vi "Shoot-Vision.vi"(11 "VisionDistance":dbl) -> (1 "Possible":bool, 2 "Speed":dbl, 3 "Angle":dbl)   [LabVIEW 2019]
panel:
  in  "maxVelocity":dbl=10.0
  in  "V2":dbl
  in  "V1":dbl
  in  "distanceToTarget":dbl
  in  "targetHight":dbl=280.0
  in  "gravityConst":dbl=9.8
  in  "angle 2":dbl=60.0
  in  "angle 1":dbl=30.0
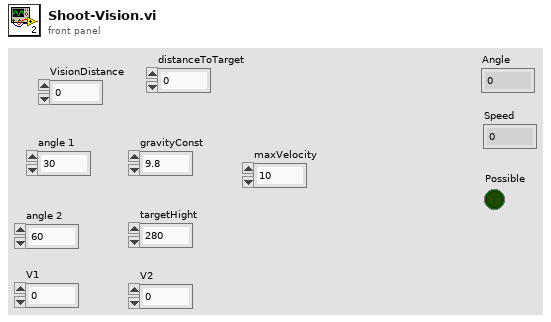
[diagram p1: front panel]
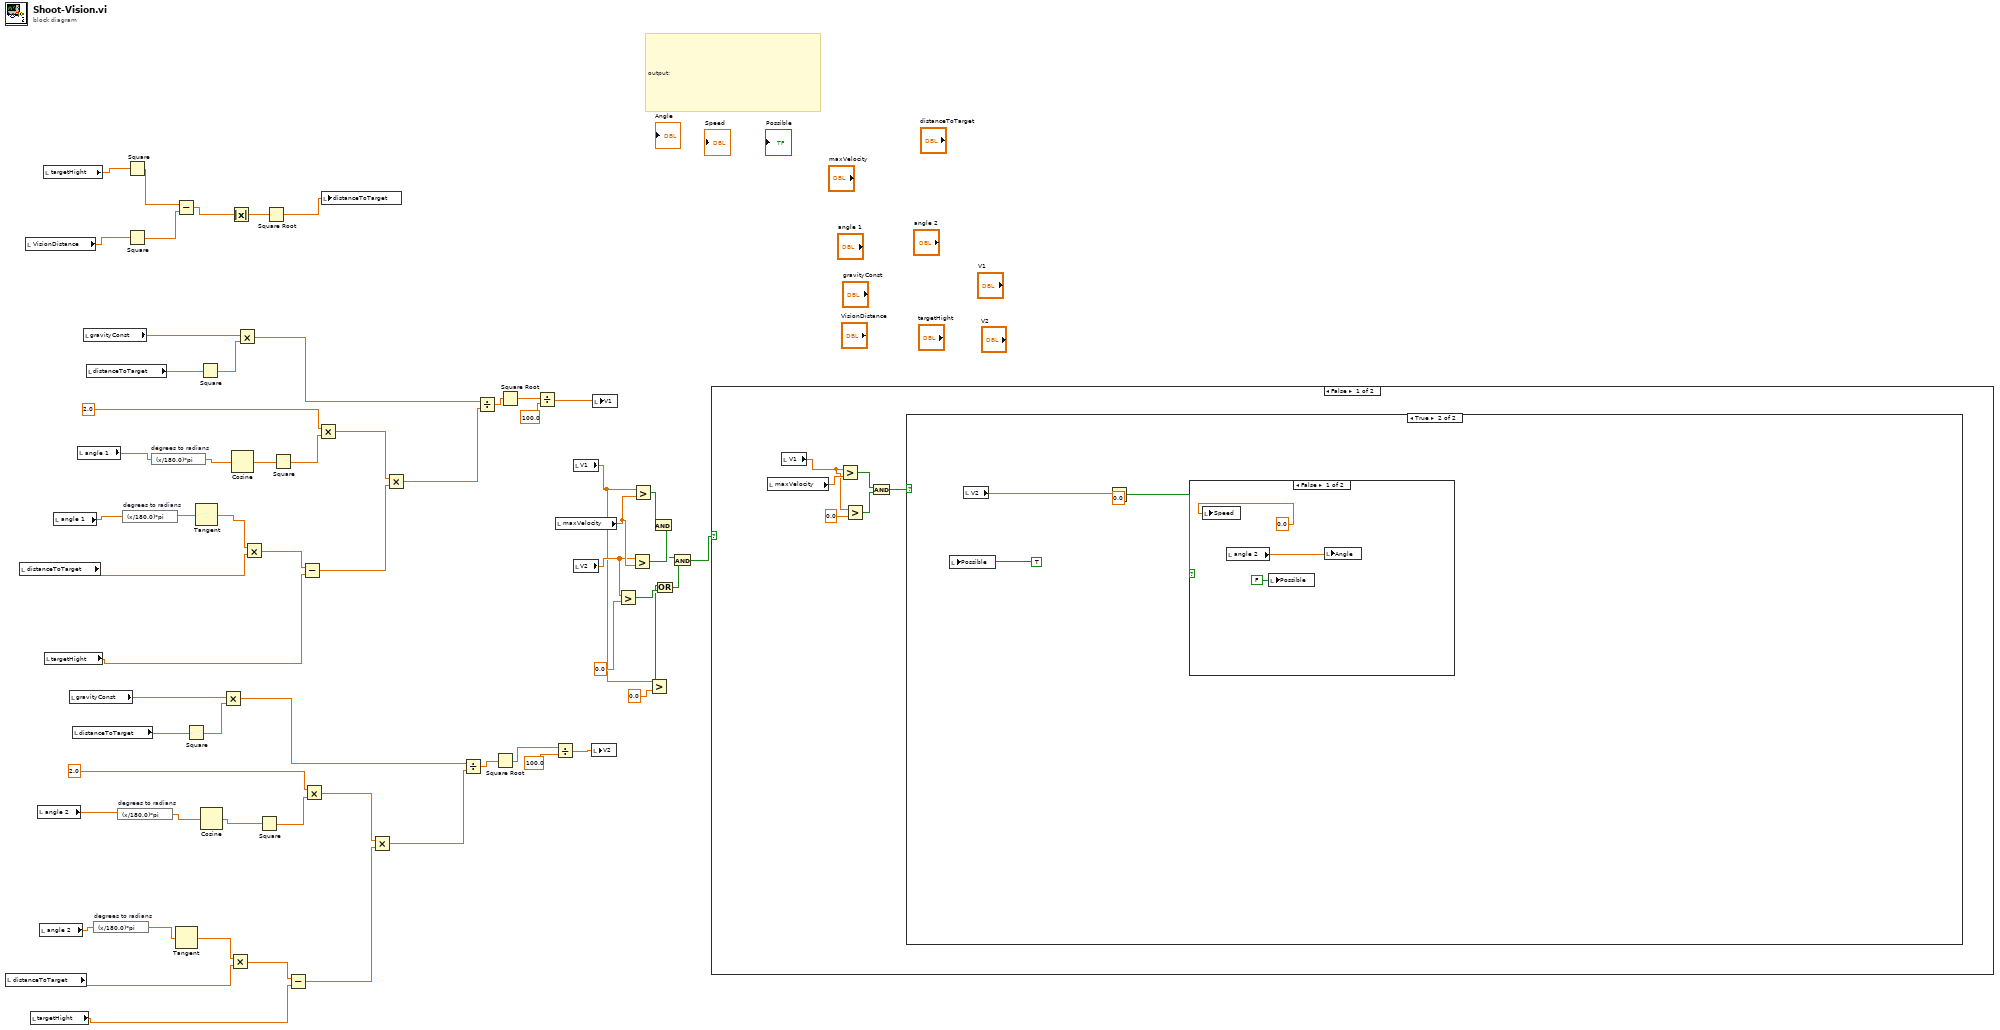
[diagram p0: block diagram]
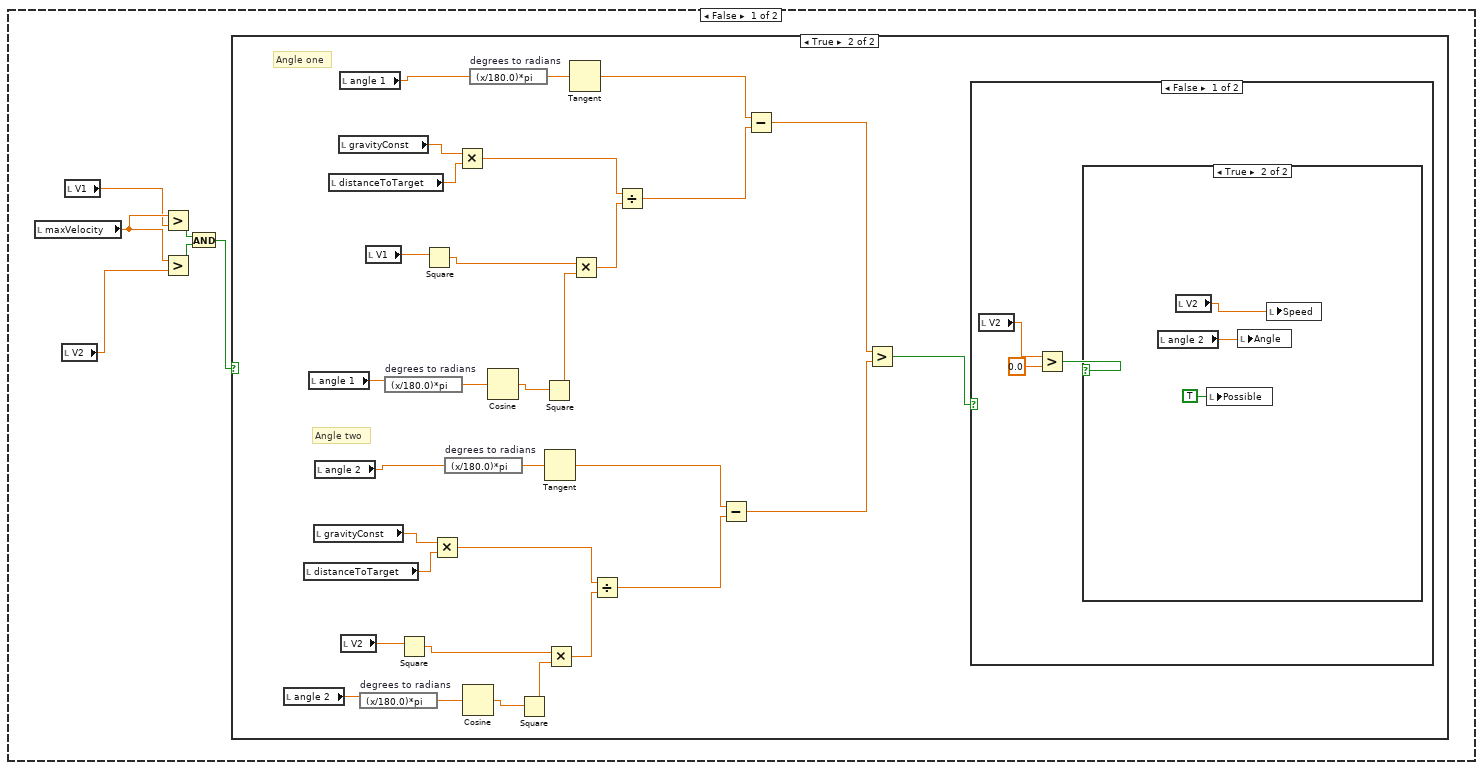
[diagram p2: hidden frame]
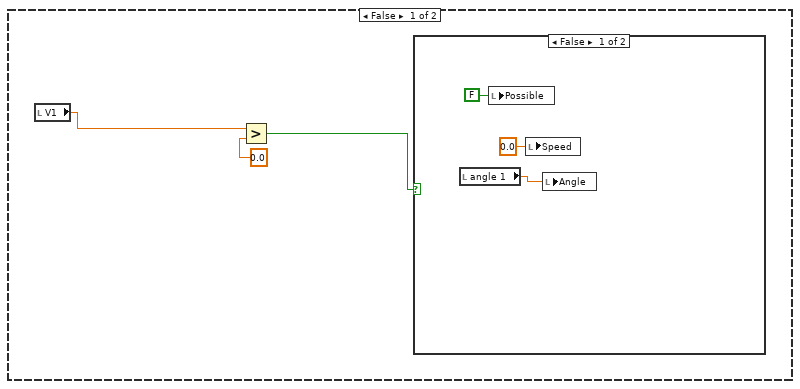
[diagram p3: hidden frame]
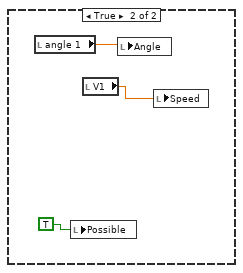
[diagram p4: hidden frame]
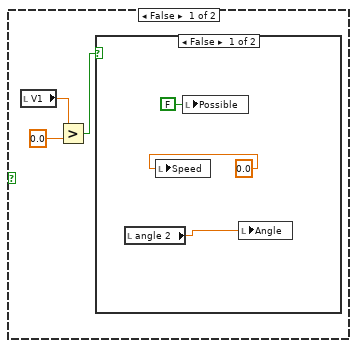
[diagram p5: hidden frame]
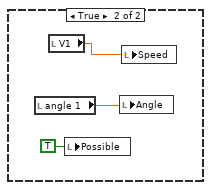
[diagram p6: hidden frame]
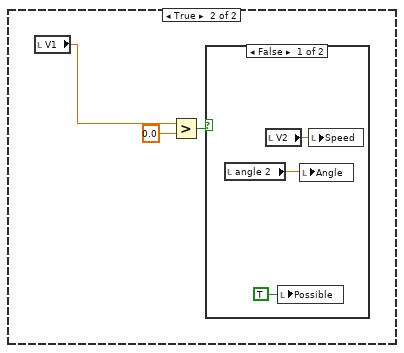
[diagram p7: hidden frame]
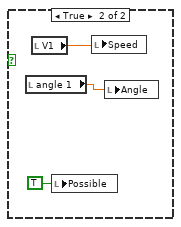
[diagram p8: hidden frame]
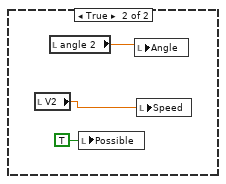
[diagram p9: hidden frame]
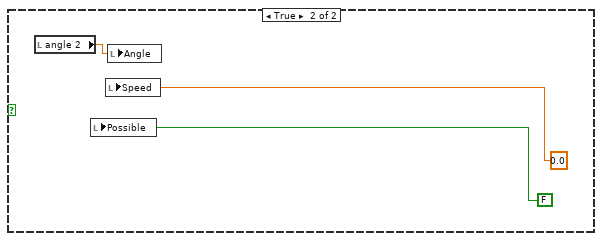
[diagram p10: hidden frame]
diagram:
  # "output:"
  n1 = local read "distanceToTarget"() -> (w42:dbl)
  n2 = local read "distanceToTarget"() -> (w51:dbl)
  n3 = local read "VisionDistance"() -> (w56:dbl)
  n4 = local read "targetHight"() -> (w44:dbl)
  n5 = local read "angle 2"() -> (w26:dbl)
  n6 = local read "angle 2"() -> (w28:dbl)
  n7 = local read "targetHight"() -> (w57:dbl)
  n8 = local read "targetHight"() -> (w49:dbl)
  n9 = local read "angle 1"() -> (w34:dbl)
  n10 = local read "gravityConst"() -> (w38:dbl)
  n11 = local read "distanceToTarget"() -> (w35:dbl)
  n12 = local read "angle 1"() -> (w29:dbl)
  n13 = local read "gravityConst"() -> (w55:dbl)
  n14 = local read "distanceToTarget"() -> (w61:dbl)
  n15 = expression code="(x/180.0)*pi" "degrees to radians"(w28) -> (w27:dbl)
  n16 = expression code="(x/180.0)*pi" "degrees to radians"(w26) -> (w25:dbl)
  n17 = expression code="(x/180.0)*pi" "degrees to radians"(w34) -> (w32:dbl)
  n18 = Square(x=w57) -> (x^2=w63:dbl)
  n19 = Square(x=w56) -> (x^2=w62:dbl)
  n20 = expression code="(x/180.0)*pi" "degrees to radians"(w29) -> (w31:dbl)
  n21 = Subtract(x=w63, y=w62) -> (x-y=w20:dbl)
  n22 = Tangent(1:w27) -> (0:w23:dbl)
  n23 = Square(x=w35) -> (x^2=w36:dbl)
  n24 = Tangent(1:w32) -> (0:w33:dbl)
  n25 = Square(x=w61) -> (x^2=w60:dbl)
  n26 = Cosine(x=w25) -> (cos(x)=w24:dbl)
  n27 = Multiply(x=w38, y=w36) -> (x*y=w37:dbl)
  n28 = Multiply(x=w23, y=w42) -> (x*y=w43:dbl)
  n29 = Absolute Value(x=w20) -> (abs(x)=w19:dbl)
  n30 = Cosine(x=w31) -> (cos(x)=w30:dbl)
  n31 = Multiply(x=w55, y=w60) -> (x*y=w58:dbl)
  n32 = Multiply(x=w33, y=w51) -> (x*y=w50:dbl)
  n33 = Square(x=w24) -> (x^2=w39:dbl)
  n34 = Square Root(x=w19) -> (sqrt(x)=w59:dbl)
  n35 = Square(x=w30) -> (x^2=w54:dbl)
  n36 = Subtract(x=w43, y=w44) -> (x-y=w45:dbl)
  n37 = Subtract(x=w50, y=w49) -> (x-y=w48:dbl)
  n38 = Multiply(x=2.0, y=w39) -> (x*y=w41:dbl)
  n39 = Multiply(x=2.0, y=w54) -> (x*y=w52:dbl)
  n40 = local write "distanceToTarget"(w59) -> ()
  n41 = Multiply(x=w41, y=w45) -> (x*y=w46:dbl)
  n42 = Multiply(x=w52, y=w48) -> (x*y=w47:dbl)
  n43 = Divide(x=w37, y=w46) -> (x/y=w2:dbl)
  n44 = Divide(x=w58, y=w47) -> (x/y=w4:dbl)
  n45 = Square Root(x=w2) -> (sqrt(x)=w1:dbl)
  n46 = Square Root(x=w4) -> (sqrt(x)=w3:dbl)
  n47 = Divide(x=w3, y=100.0) -> (x/y=w17:dbl)
  n48 = Divide(x=w1, y=100.0) -> (x/y=w15:dbl)
  n49 = local read "maxVelocity"() -> (w21:dbl)
  n50 = local read "V1"() -> (w9:dbl)
  n51 = local read "V2"() -> (w11:dbl)
  n52 = local write "V2"(w15) -> ()
  n53 = local write "V1"(w17) -> ()
  n54 = Greater?(x=w11, y=0.0) -> (0:w12:bool)
  n55 = Greater?(x=w11, y=w21) -> (0:w13:bool)
  n56 = Greater?(x=w9, y=w21) -> (0:w22:bool)
  n57 = Greater?(x=w9, y=0.0) -> (0:w8:bool)
  n58 = And(x=w22, y=w13) -> (x .and. y?=w7:bool)
  n59 = Or(x=w8, y=w12) -> (x .or. y?=w5:bool)
  n60 = And(x=w7, y=w5) -> (x .and. y?=w6:bool)
  n61 = case shown="False" w6 {
    frame False {
      n62 = local read "maxVelocity"() -> (w69:dbl)
      n63 = local read "V1"() -> (w68:dbl)
      n64 = Greater?(x=w68, y=w69) -> (0:w65:bool)
      n65 = Greater?(x=w68, y=0.0) -> (0:w64:bool)
      n66 = And(x=w65, y=w64) -> (x .and. y?=w66:bool)
      n67 = case shown="True" w66 {
        frame False {
          n68 = local read "maxVelocity"() -> (w75:dbl)
          n69 = local read "V2"() -> (w72:dbl)
          n70 = local read "V1"() -> (w71:dbl)
          n71 = Greater?(x=w75, y=w71) -> (0:w74:bool)
          n72 = Greater?(x=w75, y=w72) -> (0:w73:bool)
          n73 = And(x=w74, y=w73) -> (x .and. y?=w70:bool)
          n74 = case shown="True" w70 {
            frame False {
              n75 = local read "V1"() -> (w78:dbl)
              n76 = Greater?(x=w78, y=0.0) -> (0:w76:bool)
              n77 = case shown="False" w76 {
                frame False {
                  n78 = local read "angle 1"() -> (w80:dbl)
                  n79 = local write "Possible"(FALSE ("Possible")) -> ()
                  n80 = local write "Speed"(0.0 ("Speed")) -> ()
                  n81 = local write "Angle"(w80) -> ()
                }
                frame True {
                  n82 = local read "angle 1"() -> (w83:dbl)
                  n83 = local write "Possible"(TRUE ("Possible")) -> ()
                  n84 = local read "V1"() -> (w82:dbl)
                  n85 = local write "Angle"(w83) -> ()
                  n86 = local write "Speed"(w82) -> ()
                }
              }
            }
            frame True {
              # "Angle two"
              # "Angle one"
              n87 = local read "angle 2"() -> (w94:dbl)
              n88 = local read "distanceToTarget"() -> (w91:dbl)
              n89 = local read "angle 1"() -> (w109:dbl)
              n90 = local read "gravityConst"() -> (w90:dbl)
              n91 = local read "angle 2"() -> (w89:dbl)
              n92 = local read "distanceToTarget"() -> (w112:dbl)
              n93 = local read "gravityConst"() -> (w113:dbl)
              n94 = local read "angle 1"() -> (w114:dbl)
              n95 = local read "V2"() -> (w92:dbl)
              n96 = expression code="(x/180.0)*pi" "degrees to radians"(w94) -> (w93:dbl)
              n97 = local read "V1"() -> (w111:dbl)
              n98 = expression code="(x/180.0)*pi" "degrees to radians"(w109) -> (w110:dbl)
              n99 = Square(x=w92) -> (x^2=w96:dbl)
              n100 = Square(x=w111) -> (x^2=w107:dbl)
              n101 = Multiply(x=w90, y=w91) -> (x*y=w98:dbl)
              n102 = expression code="(x/180.0)*pi" "degrees to radians"(w89) -> (w88:dbl)
              n103 = Multiply(x=w113, y=w112) -> (x*y=w105:dbl)
              n104 = Cosine(x=w93) -> (cos(x)=w95:dbl)
              n105 = expression code="(x/180.0)*pi" "degrees to radians"(w114) -> (w115:dbl)
              n106 = Cosine(x=w110) -> (cos(x)=w108:dbl)
              n107 = Square(x=w95) -> (x^2=w97:dbl)
              n108 = Square(x=w108) -> (x^2=w106:dbl)
              n109 = Tangent(1:w88) -> (0:w100:dbl)
              n110 = Multiply(x=w96, y=w97) -> (x*y=w99:dbl)
              n111 = Tangent(1:w115) -> (0:w103:dbl)
              n112 = Multiply(x=w107, y=w106) -> (x*y=w104:dbl)
              n113 = Divide(x=w98, y=w99) -> (x/y=w101:dbl)
              n114 = Divide(x=w105, y=w104) -> (x/y=w102:dbl)
              n115 = Subtract(x=w100, y=w101) -> (x-y=w86:dbl)
              n116 = Subtract(x=w103, y=w102) -> (x-y=w87:dbl)
              n117 = Greater?(x=w87, y=w86) -> (0:w85:bool)
              n118 = case shown="False" w85 {
                frame False {
                  n119 = local read "V2"() -> (w118:dbl)
                  n120 = Greater?(x=w118, y=0.0) -> (0:w116:bool)
                  n121 = case shown="True" w116 {
                    frame False {
                      n122 = local read "V1"() -> (w121:dbl)
                      n123 = Greater?(x=w121, y=0.0) -> (0:w119:bool)
                      n124 = case shown="False" w119 {
                        frame False {
                          n125 = local read "angle 2"() -> (w122:dbl)
                          n126 = local write "Speed"(0.0 ("Speed")) -> ()
                          n127 = local write "Possible"(FALSE ("Possible")) -> ()
                          n128 = local write "Angle"(w122) -> ()
                        }
                        frame True {
                          n129 = local read "angle 1"() -> (w127:dbl)
                          n130 = local read "V1"() -> (w125:dbl)
                          n131 = local write "Possible"(TRUE ("Possible")) -> ()
                          n132 = local write "Angle"(w127) -> ()
                          n133 = local write "Speed"(w125) -> ()
                        }
                      }
                    }
                    frame True {
                      n134 = local read "angle 2"() -> (w129:dbl)
                      n135 = local read "V2"() -> (w130:dbl)
                      n136 = local write "Possible"(TRUE ("Possible")) -> ()
                      n137 = local write "Angle"(w129) -> ()
                      n138 = local write "Speed"(w130) -> ()
                    }
                  }
                }
                frame True {
                  n139 = local read "V1"() -> (w133:dbl)
                  n140 = Greater?(x=w133, y=0.0) -> (0:w131:bool)
                  n141 = case shown="False" w131 {
                    frame False {
                      n142 = local read "angle 2"() -> (w135:dbl)
                      n143 = local read "V2"() -> (w136:dbl)
                      n144 = local write "Possible"(TRUE ("Possible")) -> ()
                      n145 = local write "Angle"(w135) -> ()
                      n146 = local write "Speed"(w136) -> ()
                    }
                    frame True {
                      n147 = local read "angle 1"() -> (w138:dbl)
                      n148 = local read "V1"() -> (w139:dbl)
                      n149 = local write "Possible"(TRUE ("Possible")) -> ()
                      n150 = local write "Speed"(w139) -> ()
                      n151 = local write "Angle"(w138) -> ()
                    }
                  }
                }
              }
            }
          }
        }
        frame True {
          n152 = local write "Possible"(TRUE ("Possible")) -> ()
          n153 = local read "V2"() -> (w142:dbl)
          n154 = Greater?(x=w142, y=0.0) -> (0:w140:bool)
          n155 = case shown="False" w140 {
            frame False {
              n156 = local write "Speed"(0.0 ("Speed")) -> ()
              n157 = local read "angle 2"() -> (w145:dbl)
              n158 = local write "Possible"(FALSE ("Possible")) -> ()
              n159 = local write "Angle"(w145) -> ()
            }
            frame True {
              n160 = local read "V2"() -> (w148:dbl)
              n161 = local read "angle 2"() -> (w149:dbl)
              n162 = local write "Possible"(TRUE ("Possible")) -> ()
              n163 = local write "Angle"(w149) -> ()
              n164 = local write "Speed"(w148) -> ()
            }
          }
        }
      }
    }
    frame True {
      n165 = local read "angle 2"() -> (w151:dbl)
      n166 = local write "Possible"(FALSE ("Possible")) -> ()
      n167 = local write "Speed"(0.0 ("Speed")) -> ()
      n168 = local write "Angle"(w151) -> ()
    }
  }
